vi "Calibration FGV.vi"(10 "Calib in":T2(array[cluster]), 11 "FGV States":T1) -> (2 "Calib in 2":T2(array[cluster]))   [LabVIEW 2016]
uses:
  FGV States.ctl
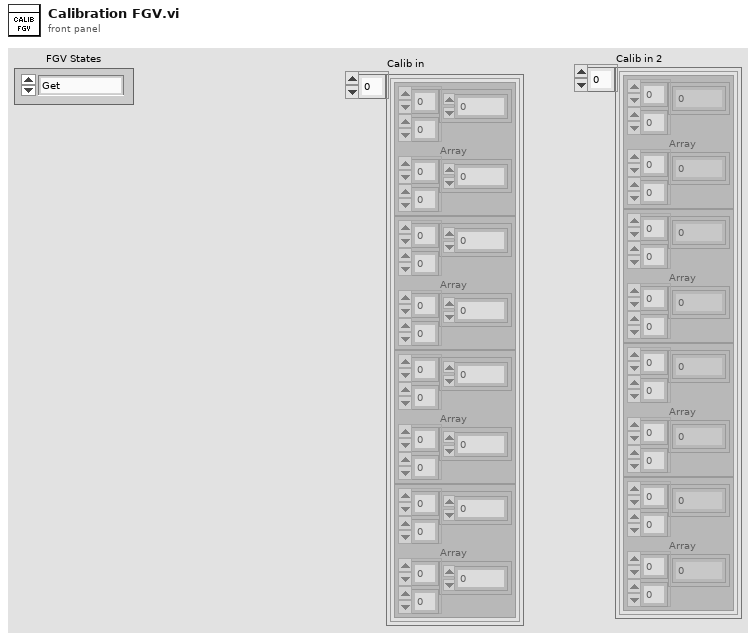
[diagram p1: front panel]
types:
  T1 = typedef "FGV States.ctl" = enum16{"Get", "Set", "Reset"}
  T2 = cluster{cluster{dbl[][], "Array":dbl[][]}, cluster{dbl[][], "Array":dbl[][]}, cluster{dbl[][], "Array":dbl[][]}, cluster{dbl[][], "Array":dbl[][]}}[]
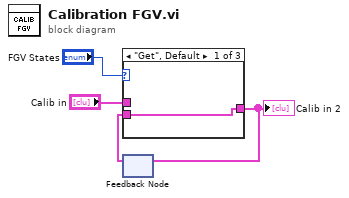
[diagram p0: block diagram]
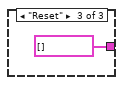
[diagram p3: hidden frame]
diagram:
  n1 = feedback #1() -> (w2:T2)  [unwired: 1 in]
  n2 = case shown="\"Get\", Default" "FGV States" {
    tunnel: "Calib in" -> [_ w6 _]
    tunnel: [w5 w6 T2 [] ("Calib in")] -> w3
    tunnel: w2 -> [w5 _ _]
    frame "Get", Default {
    }
    frame "Set" {
    }
    frame "Reset" {
    }
  }
  "Calib in 2" <- w3
  n3 = feedback-in #1(w3) -> ()
